vi "Network Steam Write Message.vi"(6 "Timeout(ms)":i32, 7 "Wait for Ack? (false)":bool, 8 "error in (no error)":errorcluster, 10 "Message":T1={"Command"="", "Arguments"=variant, " Msg Id"=-1, "Data"=""}, 11 "Model in":refnum<class "Model.lvclass">) -> (0 "error out":errorcluster, 2 "StillConnected?":bool, 3 "Model out":refnum<class "Model.lvclass">, 4 "Timed Out?":bool)   [LabVIEW 2021, in "Model.lvlib" / "Model.lvclass"]
uses:
  Model.lvclass
  Model.lvclass/Model.ctl
  <userlib>/John_Lib/Network_Streams_Connection/NetworkConnection.lvclass
  <userlib>/John_Lib/Network_Streams_Connection/NetworkCommand--Cluster.ctl
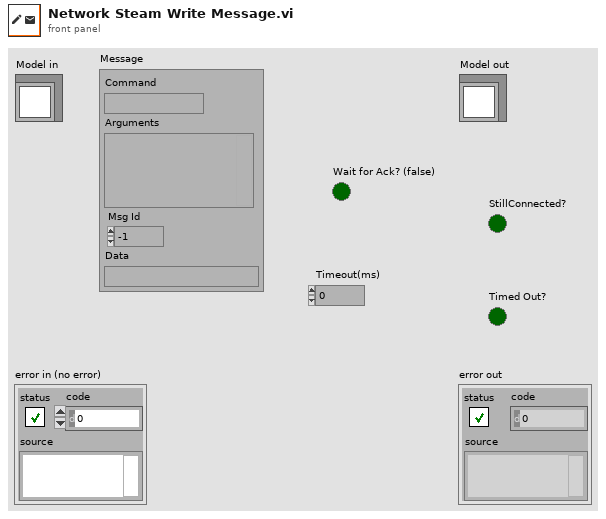
[diagram p1: front panel]
types:
  T1 = typedef "JKI_Network_Streams.lvlib/NetworkConnection.lvclass/NetworkCommand--Cluster.ctl" = cluster{"Command":string, "Arguments":variant, " Msg Id":i32, "Data":string}
  T2 = typedef "Model.lvlib/Model.lvclass/DVR.ctl" = cluster{"JKI_Network_Streams":refnum<class "NetworkConnection.lvclass">}
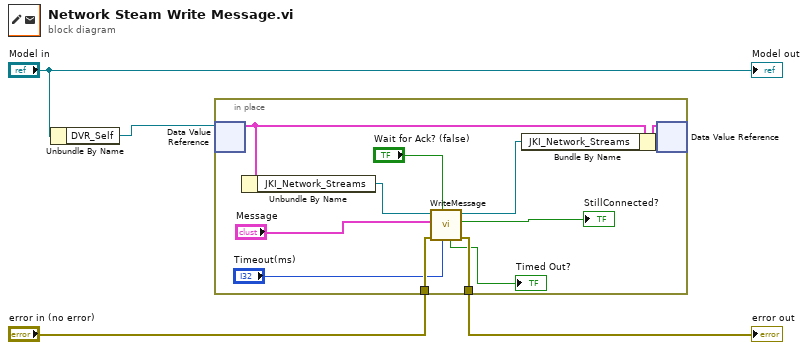
[diagram p0: block diagram]
diagram:
  n1 = Unbundle By Name("Model in") -> ("DVR_Self"=w3:refnum<data-value>)
  n2 = in-place {
    in-place-border: "error in (no error)" -> [w9]
    in-place-border: [w8] -> w1
    n3 = in-place-dvr #1(w3) -> (w15:T2)  [unwired: 1 out]
    n4 = Unbundle By Name(w15) -> ("JKI_Network_Streams"=w14:refnum<class "NetworkConnection.lvclass">)
    n5 = call <userlib>:"WriteMessage.vi"("Timeout(ms)"="Timeout(ms)", "Wait for Ack? (false)"="Wait for Ack? (false)", "error in (no error)"=w9, "Message"="Message", "NetworkConnection in"=w14) -> ("error out"=w8:errorcluster, "StillConnected?"=→"StillConnected?":bool, "NetworkConnection out"=w12:refnum<class "NetworkConnection.lvclass">, "Timed Out?"=→"Timed Out?":bool)  [unwired: 3 in]
    n6 = Bundle By Name(cluster=w15, "JKI_Network_Streams"=w12) -> (w13:T2)
    n7 = in-place-dvr #1(w13) -> ()  [unwired: 2 out]
  }
  "error out" <- w1
  "Model out" <- "Model in"
